vi "TPlot.vi"(11 "通道输入":string) -> ()   [LabVIEW 2018, in "DataDisplay.lvlib"]
uses:
  DataDisplay.lvlib
  TPlot/TPlot.lvclass
  TPlot/TPlotRef.ctl
  TypeDefine/DD_DataStream.ctl
  SubVI/DD_Parameter.vi
panel:
  in  "显示副曲线":bool
  in  "1图形选择":u16(ring) items=["位移1", "力1", "次数1", "位移2", "力2", "次数2"]
  in  "0图形选择":u16(ring) items=["位移1", "力1", "次数1", "位移2", "力2", "次数2"]
  out "波形图":waveform(dbl)[](graph)
  # "Y轴"
  # "副曲线"
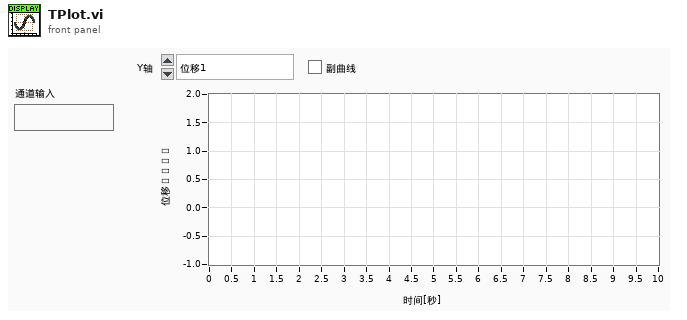
[diagram p1: front panel]
types:
  T1 = typedef "DataDisplay.lvlib/TPlot.lvclass/TPlotRef.ctl" = cluster{"rVI":refnum<vi>, "rPane":refnum<vi>, "r波形图":refnum<vi>, "r通道选择0":refnum<vi>, "r通道选择1":refnum<vi>, "r显示副曲线":refnum<vi>, "DD_数据通知器":refnum<notifier>}
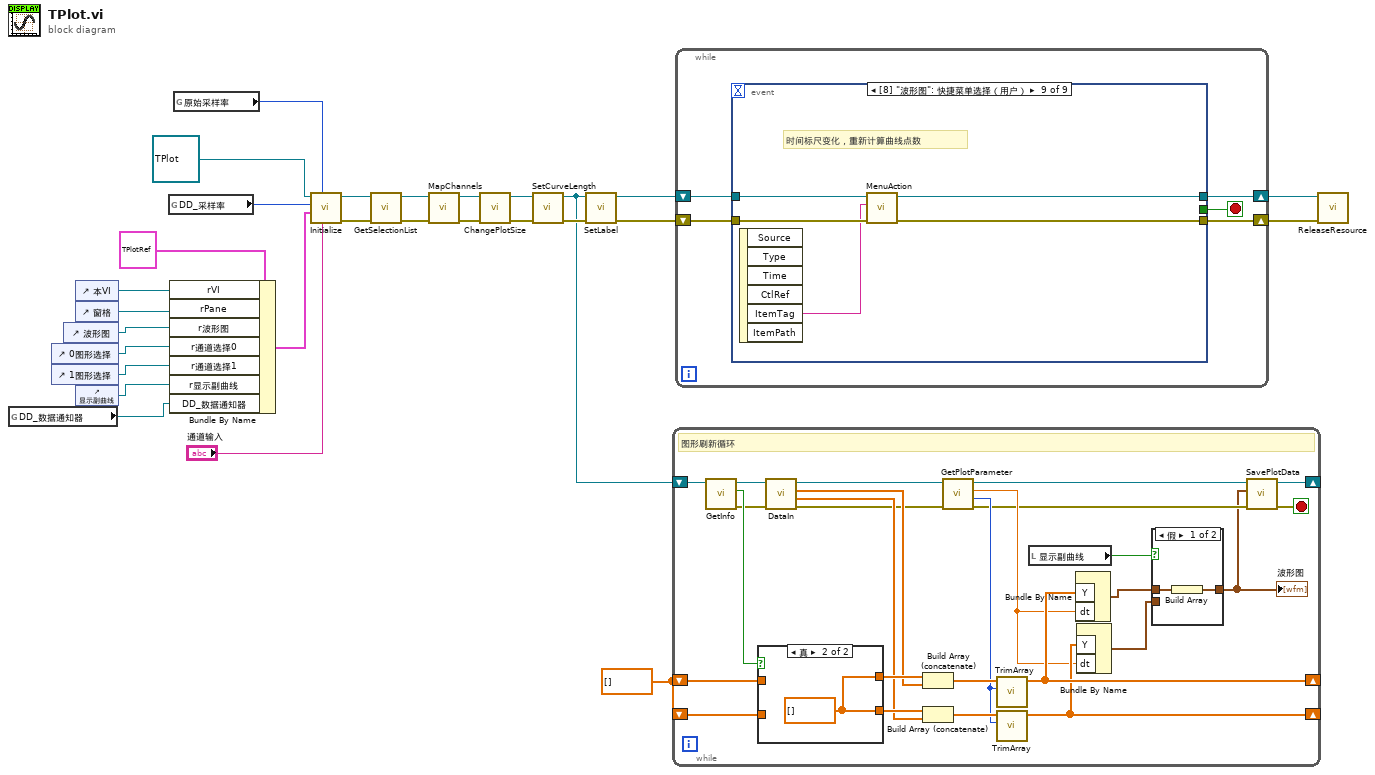
[diagram p0: block diagram]
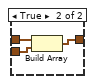
[diagram p3: hidden frame]
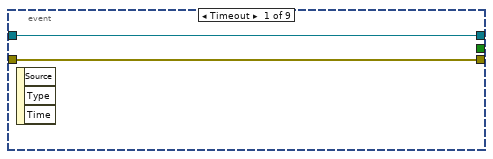
[diagram p4: hidden frame]
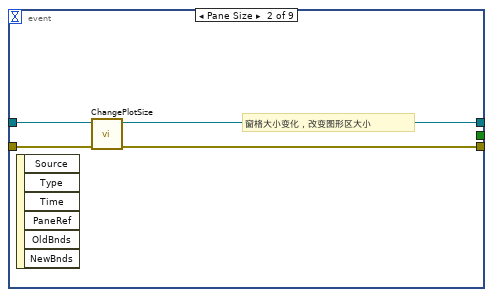
[diagram p5: hidden frame]
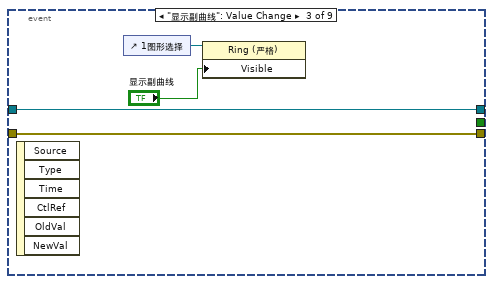
[diagram p6: hidden frame]
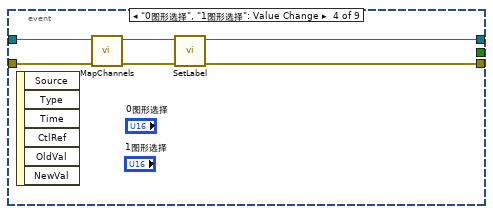
[diagram p7: hidden frame]
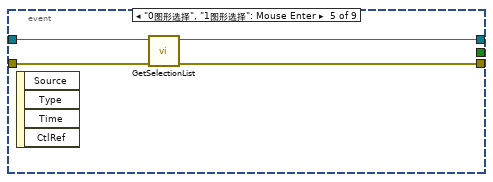
[diagram p8: hidden frame]
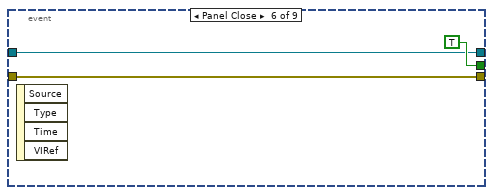
[diagram p9: hidden frame]
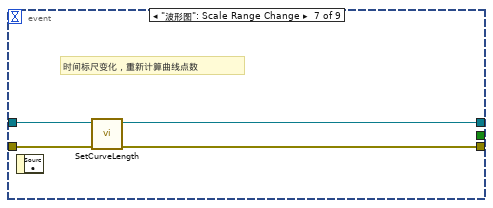
[diagram p10: hidden frame]
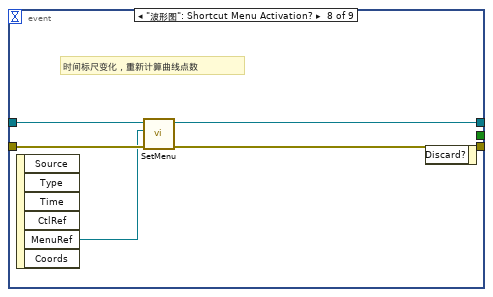
[diagram p11: hidden frame]
diagram:
  w9 = dbl[] []
  n1 = global read "DD_Parameter.vi" "DD_数据通知器"() -> (w10:refnum<notifier>)
  n2 = control-ref of="0图形选择"() -> (w22:refnum<vi>)
  n3 = control-ref of="1图形选择"() -> (w21:refnum<vi>)
  n4 = control-ref of="波形图"() -> (w23:refnum<vi>)
  n5 = control-ref of="本VI"() -> (w25:refnum<vi>)
  n6 = control-ref of="窗格"() -> (w24:refnum<vi>)
  n7 = control-ref of="显示副曲线"() -> (w20:refnum<vi>)
  n8 = global read "DD_Parameter.vi" "DD_采样率"() -> (w27:i32)
  n9 = Bundle By Name(cluster=T1 {"rVI"=refnum, "rPane"=refnum, "r波形图"=refnum, "r通道选择0"=refnum, "r通道选择1"=refnum, "r显示副曲线"=refnum, "DD_数据通知器"=refnum} ("引用"), "rVI"=w25, "rPane"=w24, "r波形图"=w23, "r通道选择0"=w22, "r通道选择1"=w21, "r显示副曲线"=w20, "DD_数据通知器"=w10) -> (w19:T1)
  n10 = global read "DD_Parameter.vi" "原始采样率"() -> (w2:i32)
  n11 = call "Initialize.vi"("通道输入"="通道输入", "原始采样率[Hz]"=w2, "引用"=w19, "显示采样率[Hz]"=w27, "TPlot 输入"=refnum<class "TPlot.lvclass"> refnum ("DataDisplay.lvlib:TPlot.lvclass")) -> ("error out"=w17:errorcluster, "TPlot 输出"=w5:refnum<class "TPlot.lvclass">)  [unwired: 5 in]
  n12 = call "GetSelectionList.vi"("error in (no error)"=w17, "TPlot 输入"=w5) -> ("error out"=w16:errorcluster, "TPlot 输出"=w18:refnum<class "TPlot.lvclass">)  [unwired: 8 in]
  n13 = call "MapChannels.vi"("error in (no error)"=w16, "TPlot 输入"=w18) -> ("error out"=w15:errorcluster, "TPlot 输出"=w4:refnum<class "TPlot.lvclass">)  [unwired: 8 in]
  n14 = call "ChangePlotSize.vi"("error in (no error)"=w15, "TPlot 输入"=w4) -> ("error out"=w13:errorcluster, "TPlot 输出"=w14:refnum<class "TPlot.lvclass">)  [unwired: 8 in]
  n15 = call "SetCurveLength.vi"("error in (no error)"=w13, "TPlot 输入"=w14) -> ("error out"=w12:errorcluster, "TPlot 输出"=w3:refnum<class "TPlot.lvclass">)  [unwired: 8 in]
  n16 = call "SetLabel.vi"("error in (no error)"=w12, "TPlot 输入"=w3) -> ("error out"=w11:errorcluster, "TPlot 输出"=w8:refnum<class "TPlot.lvclass">)  [unwired: 8 in]
  n17 = while {
    shift-right: [w54] -> _
    shift-left: w9 -> [w48]
    shift-right: [w43] -> _
    shift-left: w9 -> [w46]
    shift-right: [w30] -> _
    shift-left: w3 -> [w50]
    stop <- w32 stop-if-true
    # "图形刷新循环"
    n18 = call "GetInfo.vi"("TPlot 输入"=w50) -> ("error out"=w40:errorcluster, "通道变更"=w42:bool, "TPlot 输出"=w41:refnum<class "TPlot.lvclass">)  [unwired: 8 in]
    n19 = case shown="真" w42 {
      tunnel: w48 -> [w56 _]
      tunnel: [w56 w57] -> w47
      tunnel: w46 -> [w55 _]
      tunnel: [w55 w57] -> w45
      frame False {
      }
      frame True {
        w57 = dbl[] []
      }
    }
    n20 = call "DataIn.vi"("error in (no error)"=w40, "TPlot 输入"=w41) -> ("error out"=w37:errorcluster, "Data1"=w38:dbl[], "Data0"=w39:dbl[], "TPlot 输出"=w36:refnum<class "TPlot.lvclass">)  [unwired: 6 in]
    n21 = Build Array (concatenate)(w47, w39) -> (w53:dbl[])
    n22 = Build Array (concatenate)(w45, w38) -> (w44:dbl[])
    n23 = call "GetPlotParameter.vi"("error in (no error)"=w37, "TPlot 输入"=w36) -> ("error out"=w33:errorcluster, "曲线点数"=w35:i32, "时间间隔[S]"=w34:dbl, "TPlot 输出"=w31:refnum<class "TPlot.lvclass">)  [unwired: 6 in]
    n24 = call "TrimArray.vi"("曲线点数"=w35, "数组输入"=w53) -> ("数组输出"=w54:dbl[])  [unwired: 9 in]
    n25 = call "TrimArray.vi"("曲线点数"=w35, "数组输入"=w44) -> ("数组输出"=w43:dbl[])  [unwired: 9 in]
    n26 = local read "显示副曲线"() -> (w49:bool)
    n27 = Bundle By Name("Y"=w54, "dt"=w34) -> (w52:waveform(dbl))  [unwired: 1 in]
    n28 = Bundle By Name("Y"=w43, "dt"=w34) -> (w51:waveform(dbl))  [unwired: 1 in]
    n29 = case shown="假" w49 {
      tunnel: [w58 w62] -> w29
      tunnel: w52 -> [w59 w61]
      tunnel: w51 -> [_ w60]
      frame False {
        n30 = Build Array(w59) -> (w58:waveform(dbl)[])
      }
      frame True {
        n31 = Build Array(w61, w60) -> (w62:waveform(dbl)[])
      }
    }
    "波形图" <- w29
    n32 = call "SavePlotData.vi"("error in (no error)"=w33, "数据输入"=w29, "TPlot 输入"=w31) -> ("error out"=w32:errorcluster, "TPlot 输出"=w30:refnum<class "TPlot.lvclass">)  [unwired: 7 in]
  }
  n33 = while {
    shift-right: [w65] -> w7
    shift-left: w8 -> [w67]
    shift-right: [w64] -> w6
    shift-left: w11 -> [w66]
    stop <- w63 stop-if-true
    n34 = event shown="[8] \"波形图\": 快捷菜单选择（用户）" {
      selector: _ -> [_ _ _ _ _ _ _ _ _]
      dyn-events: _ -> [_ _ _ _ _ _ _ _ _]
      timeout: _ -> [_ _ _ _ _ _ _ _ _]
      tunnel: w67 -> [w69 w73 w75 w83 w87 w89 w94 w99 w104]
      tunnel: w66 -> [w68 w72 w74 w82 w86 w88 w93 w98 w103]
      tunnel: [w69 w71 w75 w80 w85 w89 w92 w97 w102] -> w65
      tunnel: [w68 w70 w74 w78 w84 w88 w91 w96 w101] -> w64
      tunnel: [_ _ _ _ _ TRUE _ _ _] -> w63
      event Timeout {
        n35 = event-data() -> ()  [unwired: 1 in, 3 out]
      }
      event Pane Size {
        # "窗格大小变化，改变图形区大小"
        n36 = event-data() -> ()  [unwired: 1 in, 6 out]
        n37 = call "ChangePlotSize.vi"("error in (no error)"=w72, "TPlot 输入"=w73) -> ("error out"=w70:errorcluster, "TPlot 输出"=w71:refnum<class "TPlot.lvclass">)  [unwired: 8 in]
      }
      event "显示副曲线": Value Change {
        n38 = event-data() -> ()  [unwired: 1 in, 6 out]
        n39 = control-ref of="1图形选择"() -> (w77:refnum<vi>)
        n40 = property class="Ring (严格)"(reference=w77, "Visible"="显示副曲线") -> ()  [unwired: 1 in, 2 out]
      }
      event "0图形选择", "1图形选择": Value Change {
        n41 = event-data() -> ()  [unwired: 1 in, 6 out]
        n42 = call "MapChannels.vi"("error in (no error)"=w82, "TPlot 输入"=w83) -> ("error out"=w79:errorcluster, "TPlot 输出"=w81:refnum<class "TPlot.lvclass">)  [unwired: 8 in]
        n43 = call "SetLabel.vi"("error in (no error)"=w79, "TPlot 输入"=w81) -> ("error out"=w78:errorcluster, "TPlot 输出"=w80:refnum<class "TPlot.lvclass">)  [unwired: 8 in]
      }
      event "0图形选择", "1图形选择": Mouse Enter {
        n44 = event-data() -> ()  [unwired: 1 in, 4 out]
        n45 = call "GetSelectionList.vi"("error in (no error)"=w86, "TPlot 输入"=w87) -> ("error out"=w84:errorcluster, "TPlot 输出"=w85:refnum<class "TPlot.lvclass">)  [unwired: 8 in]
      }
      event Panel Close {
        n46 = event-data() -> ()  [unwired: 1 in, 4 out]
      }
      event "波形图": Scale Range Change {
        # "时间标尺变化，重新计算曲线点数"
        n47 = event-data() -> ()  [unwired: 1 in, 1 out]
        n48 = call "SetCurveLength.vi"("error in (no error)"=w93, "TPlot 输入"=w94) -> ("error out"=w91:errorcluster, "TPlot 输出"=w92:refnum<class "TPlot.lvclass">)  [unwired: 8 in]
      }
      event "波形图": Shortcut Menu Activation? {
        # "时间标尺变化，重新计算曲线点数"
        n49 = event-data() -> ("MenuRef"=w95:refnum<k9>)  [unwired: 1 in, 5 out]
        n50 = call "SetMenu.vi"("error in (no error)"=w98, "菜单引用"=w95, "TPlot 输入"=w99) -> ("error out"=w96:errorcluster, "TPlot 输出"=w97:refnum<class "TPlot.lvclass">)  [unwired: 7 in]
        n51 = event-data() -> ()  [unwired: 2 in, 1 out]
      }
      event "波形图": Shortcut Menu Selection (User) {
        # "时间标尺变化，重新计算曲线点数"
        n52 = event-data() -> ("ItemTag"=w100:string)  [unwired: 1 in, 5 out]
        n53 = call "MenuAction.vi"("error in (no error)"=w103, "项标识符"=w100, "TPlot 输入"=w104) -> ("error out"=w101:errorcluster, "TPlot 输出"=w102:refnum<class "TPlot.lvclass">)  [unwired: 7 in]
      }
    }
  }
  n54 = call "ReleaseResource.vi"("error in (no error)"=w6, "TPlot 输入"=w7) -> ()  [unwired: 8 in, 2 out]
